vi "FGGA_Dry_Cal.vi"(6 "H2O":dbl, 9 "CO2_Wet":dbl, 11 "CH4_Wet":dbl) -> (1 "CO2_Dry":dbl, 3 "CH4_Dry":dbl)   [LabVIEW 2014]
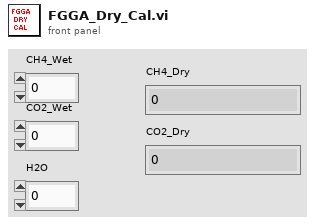
[diagram p1: front panel]
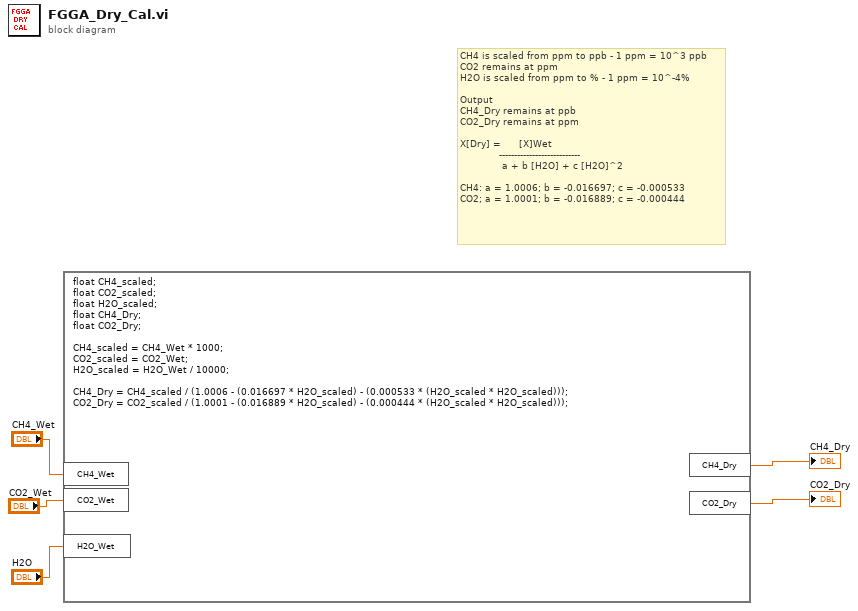
[diagram p0: block diagram]
diagram:
  # "CH4 is scaled from ppm to ppb - 1 ppm = 10^3 ppb\nCO2 remains at ppm\nH2O is scaled from ppm to % - 1 ppm = 10^-4%\n\nOutput\nCH4_Dry remains at ppb\nCO2_Dry remains at ppm\n\nX[Dry] =      [X]Wet\n             ---------------------------\n              a + b [H2O] + c [H2O]^2\n\nCH4: a = 1.0006; b = -0.016697; c = -0.000533\nCO2; a = 1.0001; b = -0.016889; c = -0.000444"
  n1 = formula code="float CH4_scaled;\nfloat CO2_scaled;\nfloat H2O_scaled;\nfloat CH4_Dry;\nfloat CO2_Dry;\n\nCH4_scaled = CH4_Wet * 1000;\nCO2_scaled = CO2_Wet;\nH2O_scaled = H2O_Wet / 10000;\n\nCH4_Dry = CH4_scaled / (1.0006 - (0.016697 * H2O_scaled) - (0.000533 * (H2O_scaled * H2O_scaled)));\nCO2_Dry = CO2_scaled / (1.0001 - (0.016889 * H2O_scaled) - (0.000444 * (H2O_scaled * H2O_scaled)));"("CH4_Wet"="CH4_Wet", "CO2_Wet"="CO2_Wet", "H2O_Wet"="H2O") -> ("CH4_Dry"=→"CH4_Dry":dbl, "CO2_Dry"=→"CO2_Dry":dbl)
